vi "Basic Accuracy Parameter2.vi"(0 "VISA resource name":refnum<visa-resource-name>, 7 "Impedance Z (10m)":dbl=0.01 min=0.01 max=100000000.0 format="%^.2e", 11 "error in (no error)":errorcluster) -> (2 "Kbb":dbl format="%^.2e", 3 "Kaa":dbl format="%^.2e", 4 "VISA resource name out":refnum<visa-resource-name>, 6 "Ka":dbl format="%.3f", 8 "Kb":dbl format="%^.2e", 10 "Kc":dbl format="%^.2e", 14 "Kd":dbl format="%^.2e", 15 "error out":errorcluster)   [LabVIEW 2015, in "Agilent 428X Series.lvlib"]
doc: "This Vi is to calculate all different K parameters. \n\nDisclaimer: All accuracy calculation VI's are not part of the original \n driver. They are provided for supplementry purpose only.\n If user desires very high accuracy data, please do or \n check the calculation seperately."
uses:
  <instrlib>/Agilent 428X Series/Agilent 428X Series.lvlib
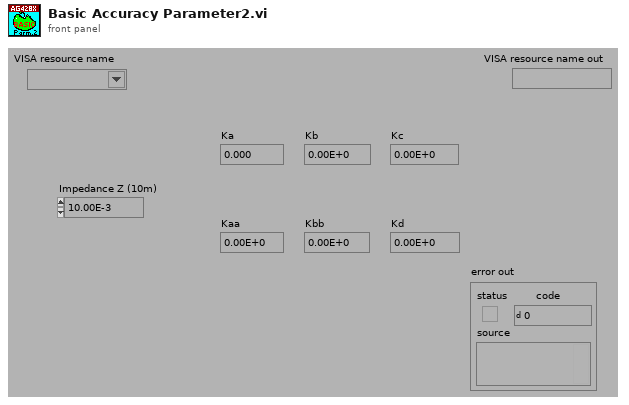
[diagram p1: front panel]
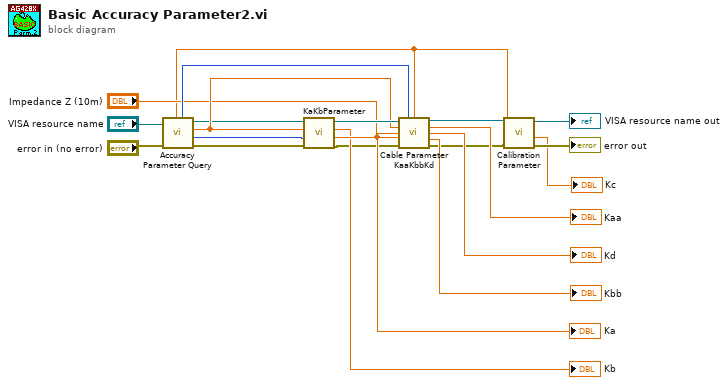
[diagram p0: block diagram]
diagram:
  n1 = call <instrlib>:"Accuracy Parameter Query.vi"("error in (no error)"="error in (no error)", "VISA resource name"="VISA resource name") -> ("error out"=w14:errorcluster, "Time Integration"=w1:u8, "Voltage Level"=w17:dbl, "VISA resource name out"=w15:refnum<visa-resource-name>, "Cable Length"=w16:i16, "Frequency"=w2:dbl)  [unwired: 4 in]
  n2 = call <instrlib>:"KaKbParameter.vi"("error in (no error)"=w14, "Integ Time (0: Short)"=w1, "Voltage Level (1.0)"=w17, "VISA resource name"=w15) -> ("error out"=w4:errorcluster, "Ka"=w18:dbl, "Kb"=→"Kb":dbl, "VISA resource name out"=w19:refnum<visa-resource-name>)  [unwired: 4 in]
  "Ka" <- w18
  n3 = call <instrlib>:"Cable Parameter KaaKbbKd.vi"("VISA resource name"=w19, "Cable Length (0:0)"=w16, "Frequency (20)"=w2, "Voltage Level (1.0)"=w17, "Impedance Z (10m)"="Impedance Z (10m)", "Ka"=w18, "error in (no error)"=w4) -> ("VISA resource name out"=w3:refnum<visa-resource-name>, "Kaa"=→"Kaa":dbl, "Kd"=→"Kd":dbl, "Kbb"=→"Kbb":dbl, "error out"=w9:errorcluster)  [unwired: 4 in]
  n4 = call <instrlib>:"Calibration Parameter.vi"("error in (no error)"=w9, "Frequency (20)"=w2, "VISA resource name"=w3) -> ("error out"=→"error out":errorcluster, "Kc"=→"Kc":dbl, "VISA resource name out"=→"VISA resource name out":refnum<visa-resource-name>)  [unwired: 6 in]
